vi "New Client.vi"(6 "Client":refnum<k5>, 8 "error in (no error)":errorcluster, 9 "Port":u16, 10 "Address":string, 11 "Messaging Server Module in":refnum<class "Messaging Server Module.lvclass">) -> (0 "error out":errorcluster, 3 "Messaging Server Module out":refnum<class "Messaging Server Module.lvclass">)   [LabVIEW 2020, in "Volatus.lvlib" / "Messaging Server Module.lvclass"]
uses:
  Messaging Server Module.lvclass
  Messaging Server Module.lvclass/Messaging Server Module.ctl
  Messaging Client/Messaging Server Client.lvclass
  Volatus.lvlib
  MessageQ/MessageQ.lvclass
  Msg Client State.ctl
  Client Info.ctl
  lv-vecto/Vecto/proto/TcpClientInfo/Data.ctl
  lv-vecto/Vecto/proto/TcpClientInfo/TcpClientInfo.lvlib
  C:/dev/lv20CE/relink/lv-volatus/Volatus/Module/Module.lvclass
  C:/dev/lv20CE/relink/lv-volatus/Volatus/Messaging Server Module/Messaging Server Module.lvclass
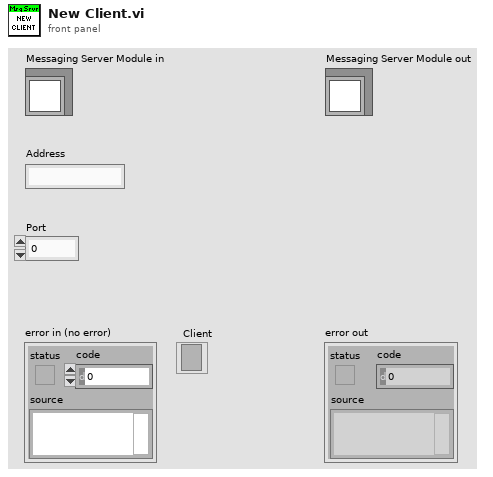
[diagram p1: front panel]
types:
  T1 = typedef "Volatus.lvlib/Msg Client State.ctl" = enum16{"Unknown", "Handshake", "Connected", "Closing"}
  T2 = typedef "Volatus.lvlib/Messaging Server Module.lvclass/Client Info.ctl" = cluster{"MsgQ":refnum<class "MessageQ.lvclass">, "Address":string, "Port":u16, "Client State":T1, "Last Update":dbl, "TCP":refnum<k5>, "Details":T3}
  T3 = typedef "TcpClientInfo.lvlib/Data.ctl" = cluster{"node_id":u32, "node_name":string, "app_version":string, "config_version":string, "config_hash":string, "node_alias":string, "address":string}
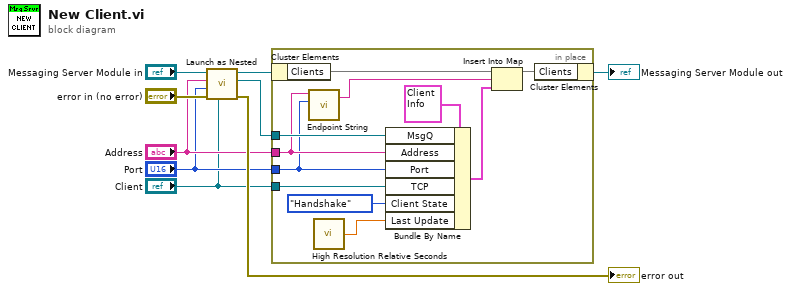
[diagram p0: block diagram]
diagram:
  n1 = call "Launch as Nested.vi"("Client"="Client", "error in (no error)"="error in (no error)", "Port"="Port", "Address"="Address", "Parent in"="Messaging Server Module in") -> ("error out"=→"error out":errorcluster, "MessageQ"=w5:refnum<class "MessageQ.lvclass">, "Parent"=w6:refnum<class "Messaging Server Module.lvclass">)  [unwired: 4 in]
  n2 = in-place {
    in-place-border: w5 -> [w15]
    in-place-border: "Address" -> [w14]
    in-place-border: "Port" -> [w12]
    in-place-border: "Client" -> [w10]
    n3 = in-place-cluster #1(w6) -> ("Clients"=w20:map{string, T2})
    n4 = call "Endpoint String.vi"("Port"=w12, "Address"=w14) -> ("Endpoint"=w19:string)  [unwired: 3 in]
    n5 = call <vilib>:"High Resolution Relative Seconds.vi"() -> ("relative seconds"=w11:dbl)
    n6 = Bundle By Name(cluster=T2 {"MsgQ"=refnum, "Address"="", "Port"=0, "Client State"=enum."Unknown", "Last Update"=0.0, "TCP"=refnum, "Details"={"node_id"=0, "node_name"="", "app_version"="", "config_version"="", "config_hash"="", "node_alias"="", "address"=""}} ("value"), "MsgQ"=w15, "Address"=w14, "Port"=w12, "TCP"=w10, "Client State"=Msg_Client_State."Handshake", "Last Update"=w11) -> (w17:T2)
    n7 = Insert Into Map(map in=w20, key=w19, value=w17) -> (map out=w16:map{string, T2})  [unwired: 2 out]
    n8 = in-place-cluster #1("Clients"=w16) -> (→"Messaging Server Module out":refnum<class "Messaging Server Module.lvclass">)
  }
